vi "Destroy Events.vi"(8 "error in (no error)":errorcluster, 11 "DLP2 in":refnum<class "DLP2.lvclass">) -> (0 "error out":errorcluster, 3 "DLP2 out":refnum<class "DLP2.lvclass">)   [LabVIEW 2022 SP3, in "DLP2.lvclass"]
doc: "Developed by Kevin Thompson\nkevin@thompsonengineering.net\n\nCopyright 2018\nThompson Engineering, LLC"
uses:
  DLP2.lvclass
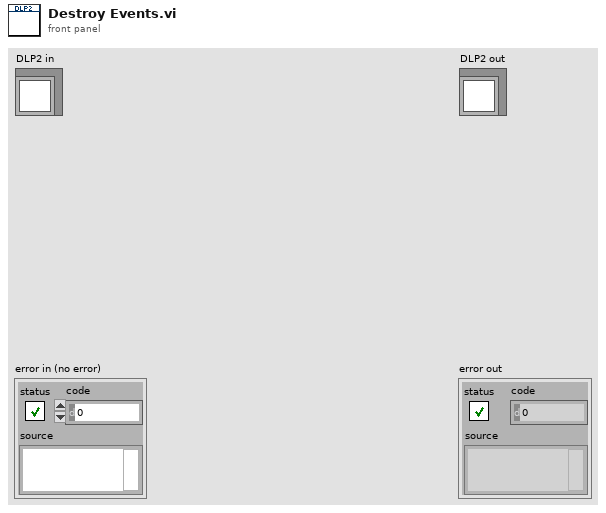
[diagram p1: front panel]
types:
  T1 = typedef "DLP2.lvclass/Public Events--cluster.ctl" = cluster{"Temp01.AsyncCmd Event":refnum<user-event>, "Temp01.AsyncMsg Event":refnum<user-event>, "stop process":refnum<user-event>, "API Incoming Event":refnum<user-event>, "API Executed Event":refnum<user-event>, "API Return Event":refnum<user-event>}
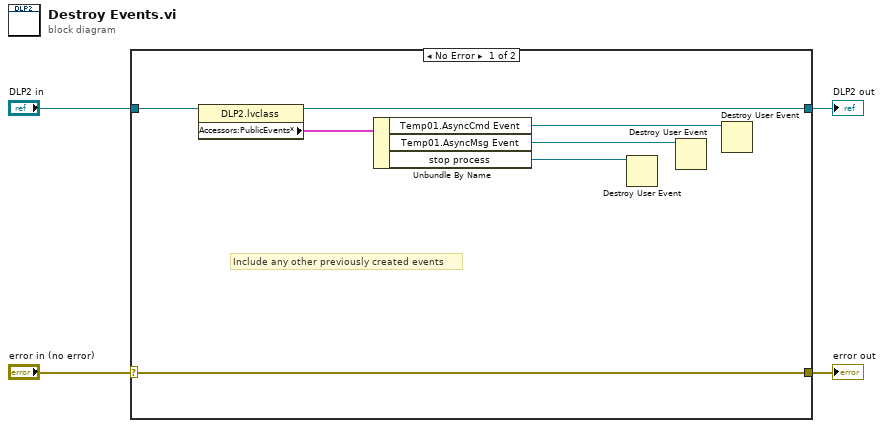
[diagram p0: block diagram]
diagram:
  n1 = case shown="No Error" "error in (no error)" {
    selector: "error in (no error)" -> [w7 w13]
    tunnel: [w7 w13] -> w3
    tunnel: [w10 w12] -> w1
    tunnel: "DLP2 in" -> [w11 w12]
    frame No Error {
      # "Include any other previously created events"
      n2 = property class="DLP2.lvclass"(reference=w11) -> (reference out=w10:refnum<class "DLP2.lvclass">, "Accessors:PublicEvents*"=w9:T1)  [unwired: 1 in, 1 out]
      n3 = Unbundle By Name(w9) -> ("Temp01.AsyncCmd Event"=w8:refnum<user-event>, "Temp01.AsyncMsg Event"=w6:refnum<user-event>, "stop process"=w5:refnum<user-event>)
      n4 = Destroy User Event(user event=w5) -> ()  [unwired: 1 in, 1 out]
      n5 = Destroy User Event(user event=w6) -> ()  [unwired: 1 in, 1 out]
      n6 = Destroy User Event(user event=w8) -> ()  [unwired: 1 in, 1 out]
    }
    frame Error {
    }
  }
  "error out" <- w3
  "DLP2 out" <- w1
